vi "LockinDAQ.Simulate Noisy AI.vi"(6 "Waveguide Cluster":T1={"Vsource Index"=0, "Vsg Index"=1, "V+"=0, "V-"=0}, 8 "error in (no error)":errorcluster, 10 "AI []":waveform(dbl)[](array[waveform]), 11 "LockinDAQ":refnum<class "LockinDAQ.lvclass">) -> (0 "error out":errorcluster, 2 "Noisy AI []":waveform(dbl)[](array[waveform]), 3 "LockinDAQ out":refnum<class "LockinDAQ.lvclass">)   [LabVIEW 2016, in "LockinDAQ.lvclass"]
uses:
  LockinDAQ.lvclass
  Waveguide Model/Waveguide Model--Cluster.ctl
  LockinDAQ.lvclass/LockinDAQ.ctl
  <vilib>/Analysis/2dsp.llb/Real FFT.vi
  <vilib>/Analysis/2dsp.llb/Inverse Real FFT.vi
  <vilib>/measure/NI_MABase.lvlib
  <vilib>/Analysis/NI_AALPro.lvlib
panel:
  in  "Noise Cluster":T2={"1/f vs. Uniform "=1.0, "60Hz Amplitude"=0.005, "Gauss/Unif %"=0.5, "Noise Amp"=0.005}
  out "Signal Graph":waveform(dbl)[](graph)
  out "Noisy Signal Graph":waveform(dbl)[](graph)
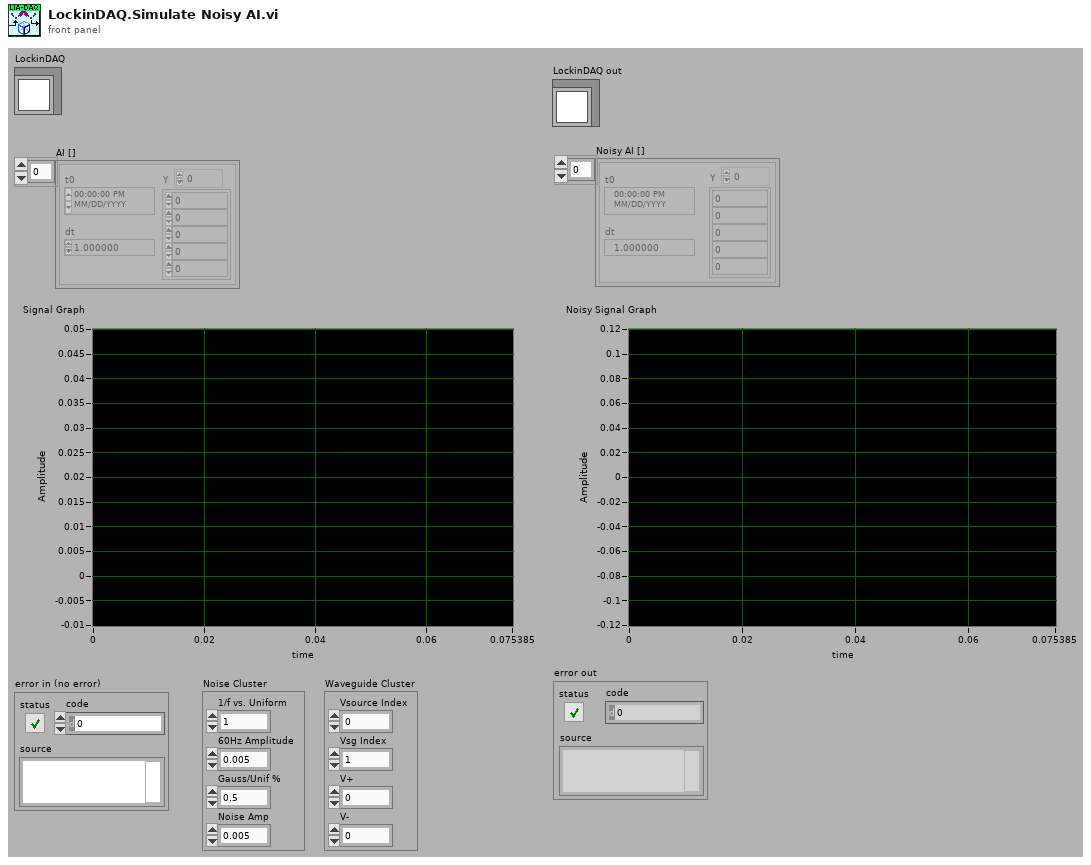
[diagram p1: front panel]
types:
  T1 = typedef "LockinDAQ.lvclass/Waveguide Model--Cluster.ctl" = cluster{"Vsource Index":i32, "Vsg Index":i32, "V+":i32, "V-":i32}
  T2 = cluster{"1/f vs. Uniform ":dbl, "60Hz Amplitude":dbl, "Gauss/Unif %":dbl, "Noise Amp":dbl}
  T3 = typedef "LockinDAQ.lvclass/Sampling.ctl" = cluster{"Fs":dbl, "#s":i32}
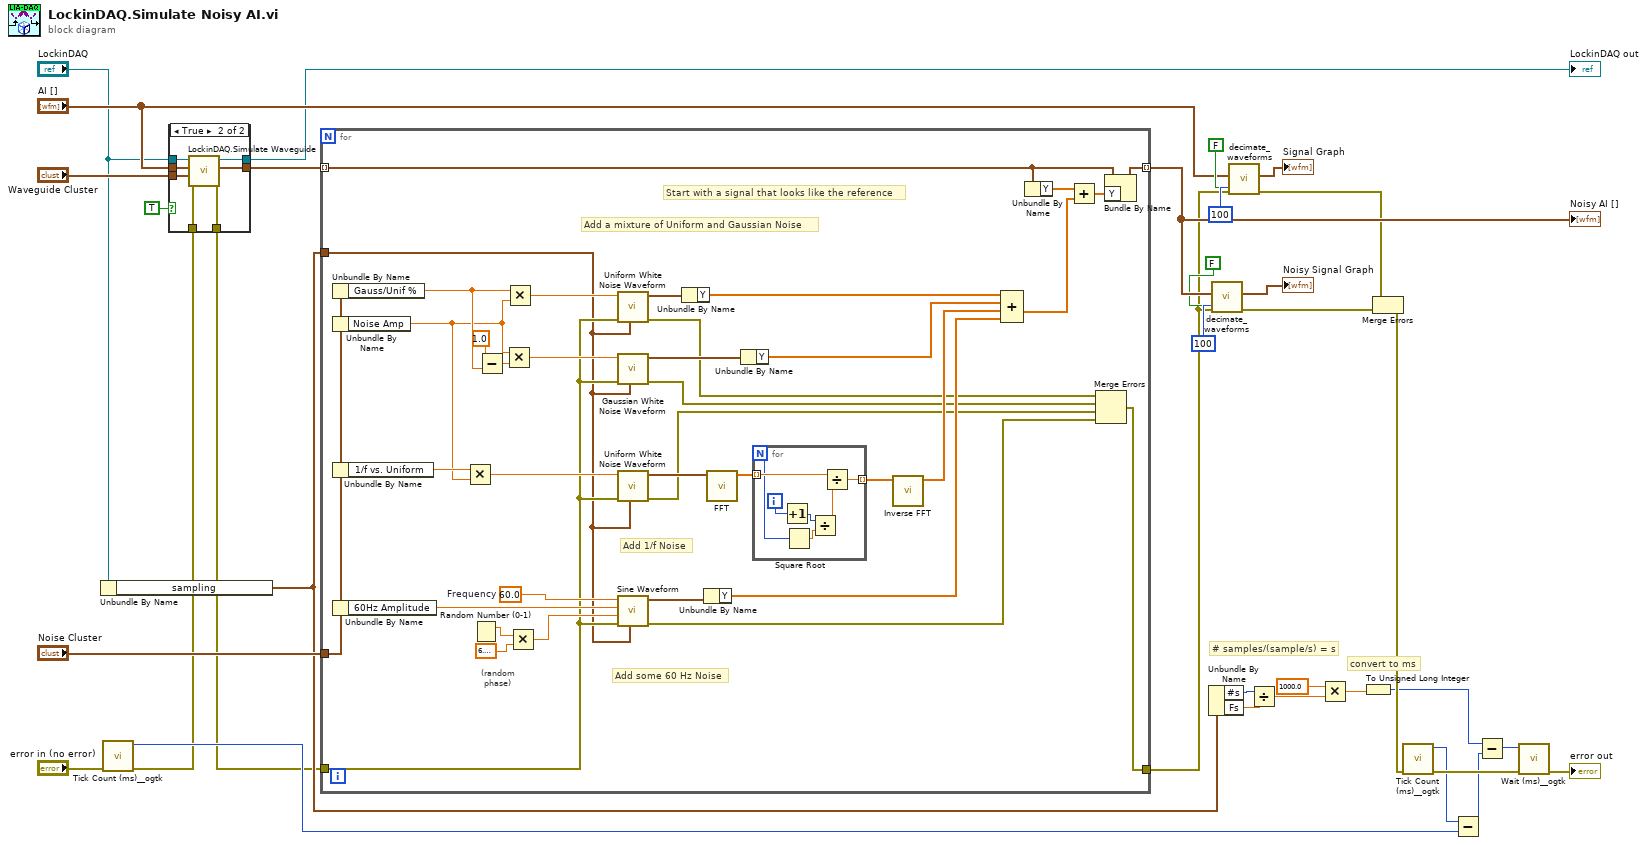
[diagram p0: block diagram]
diagram:
  # "convert to ms"
  # "# samples/(sample/s) = s"
  n1 = Unbundle By Name("LockinDAQ") -> ("sampling"=w12:T3)
  n2 = call <userlib>:"Tick Count (ms)__ogtk.vi"("error in (no error)"="error in (no error)") -> ("error out"=w10:errorcluster, "millisecond timer value"=w24:u32)  [unwired: 9 in]
  n3 = case shown="True" TRUE {
    tunnel: w10 -> [w36 w44]
    tunnel: [w36 w43] -> w9
    tunnel: [w35 w42] -> w6
    tunnel: "Waveguide Cluster" -> [_ w41]
    tunnel: "AI []" -> [w35 w40]
    tunnel: "LockinDAQ" -> [w37 w39]
    tunnel: [w37 w38] -> w2
    frame False {
    }
    frame True {
      n4 = call "LockinDAQ.Simulate Waveguide.vi"("error in (no error)"=w44, "Waveguide Cluster"=w41, "AO []"=w40, "LockinDAQ"=w39) -> ("error out"=w43:errorcluster, "AI []"=w42:waveform(dbl)[], "LockinDAQ out"=w38:refnum<class "LockinDAQ.lvclass">)  [unwired: 5 in]
    }
  }
  "LockinDAQ out" <- w2
  n5 = for {
    tunnel: "Noise Cluster" -> [w60]
    tunnel: w12 -> [w49]
    tunnel: w6 -> [w46] mode=indexing
    tunnel: [w50] -> w33 mode=indexing
    tunnel: w9 -> [w54]
    tunnel: [w51] -> w29
    w55 = 60.0  # Frequency
    # "Start with a signal that looks like the reference"
    # "Add 1/f Noise"
    # "(random\n phase)"
    # "Add some 60 Hz Noise"
    # "Add a mixture of Uniform and Gaussian Noise"
    n6 = Unbundle By Name(w60) -> ("Gauss/Unif %"=w65:dbl)
    n7 = Unbundle By Name(w60) -> ("Noise Amp"=w45:dbl)
    n8 = Unbundle By Name(w60) -> ("1/f vs. Uniform"=w64:dbl)
    n9 = Unbundle By Name(w60) -> ("60Hz Amplitude"=w63:dbl)
    n10 = Multiply(x=w64, y=w45) -> (x*y=w71:dbl)
    n11 = Random Number (0-1)() -> (number: 0 to 1=w75:dbl)
    n12 = Subtract(x=1.0, y=w65) -> (x-y=w78:dbl)
    n13 = Multiply(x=w45, y=w78) -> (x*y=w59:dbl)
    n14 = Multiply(x=w65, y=w45) -> (x*y=w58:dbl)
    n15 = Multiply(x=w75, y=6.283185307179586) -> (x*y=w57:dbl)
    n16 = call <vilib>:"Uniform White Noise Waveform.vi"("sampling info"=w49, "error in (no error)"=w54, "amplitude"=w58) -> ("error out"=w47:errorcluster, "signal out"=w79:waveform(dbl))  [unwired: 7 in]
    n17 = call <vilib>:"Gaussian White Noise Waveform.vi"("sampling info"=w49, "error in (no error)"=w54, "standard deviation"=w59) -> ("error out"=w48:errorcluster, "signal out"=w80:waveform(dbl))  [unwired: 7 in]
    n18 = call <vilib>:"Uniform White Noise Waveform.vi"("sampling info"=w49, "error in (no error)"=w54, "amplitude"=w71) -> ("error out"=w53:errorcluster, "signal out"=w70:waveform(dbl))  [unwired: 7 in]
    n19 = call <vilib>:"Sine Waveform.vi"("sampling info"=w49, "error in (no error)"=w54, "phase"=w57, "amplitude"=w63, "frequency"=w55) -> ("error out"=w52:errorcluster, "signal out"=w74:waveform(dbl))  [unwired: 5 in]
    n20 = Unbundle By Name(w79) -> ("Y"=w73:dbl[])
    n21 = Unbundle By Name(w74) -> ("Y"=w69:dbl[])
    n22 = call-poly <vilib>:"FFT.vi"("X"=w70) -> ("FFT {X}"=w56:cdb[])  [unwired: 9 in, 1 out]
    n23 = Unbundle By Name(w80) -> ("Y"=w66:dbl[])
    n24 = for {
      N -> [w84]
      tunnel: [w87] -> w72 mode=indexing
      tunnel: w56 -> [w86] mode=indexing
      i -> [w85]
      n25 = Increment(x=w85) -> (x+1=w82:i32)
      n26 = Square Root(x=w84) -> (sqrt(x)=w83:dbl)
      n27 = Divide(x=w82, y=w83) -> (x/y=w81:dbl)
      n28 = Divide(x=w86, y=w81) -> (x/y=w87:cdb)
    }
    n29 = call-poly <vilib>:"Inverse FFT.vi"("FFT {X}"=w72) -> ("X"=w68:dbl[])  [unwired: 9 in, 1 out]
    n30 = Compound Arithmetic op=ADD(w73, w66, w68, w69) -> (w67:dbl[])
    n31 = Unbundle By Name(w46) -> ("Y"=w62:dbl[])
    n32 = Add(x=w62, y=w67) -> (x+y=w61:dbl[])
    n33 = Merge Errors(w47, w48, w53, w52) -> (w51:errorcluster)
    n34 = Bundle By Name(cluster=w46, "Y"=w61) -> (w50:waveform(dbl))
  }
  "Noisy AI []" <- w33
  n35 = Unbundle By Name(w12) -> ("#s"=w14:i32, "Fs"=w15:dbl)
  n36 = call "decimate_waveforms.vi"("decimating factor"=100, "averaging"=FALSE, "error in (no error)"=w29, "WFM"=w33) -> ("error out"=w28:errorcluster, "WFM out"=→"Noisy Signal Graph":waveform(dbl)[])  [unwired: 6 in]
  n37 = call "decimate_waveforms.vi"("decimating factor"=100, "averaging"=FALSE, "error in (no error)"=w29, "WFM"="AI []") -> ("error out"=w26:errorcluster, "WFM out"=→"Signal Graph":waveform(dbl)[])  [unwired: 6 in]
  n38 = Divide(x=w14, y=w15) -> (x/y=w18:dbl)
  n39 = Multiply(x=1000.0, y=w18) -> (x*y=w17:dbl)
  n40 = To Unsigned Long Integer(number=w17) -> (unsigned 32bit integer=w13:u32)
  n41 = Merge Errors(w26, w28) -> (w25:errorcluster)
  n42 = call <userlib>:"Tick Count (ms)__ogtk.vi"("error in (no error)"=w25) -> ("error out"=w23:errorcluster, "millisecond timer value"=w19:u32)  [unwired: 9 in]
  n43 = Subtract(x=w19, y=w24) -> (x-y=w20:u32)
  n44 = Subtract(x=w13, y=w20) -> (x-y=w21:u32)
  n45 = call <userlib>:"Wait (ms)__ogtk.vi"("error in (no error)"=w23, "milliseconds to wait"=w21) -> ("error out"=→"error out":errorcluster)  [unwired: 8 in, 1 out]
